vi "Starting Point.vi"() -> ()   [LabVIEW 2017]
uses:
  <vilib>/Analysis/baseanly.llb/Real A x B.vi
  <vilib>/Analysis/NI_AALBase.lvlib
  <vilib>/picture/3D Picture Control/NI_3D Picture Control.lvlib
panel:
  out "3D Picture":refnum<vi>(3d-picture)
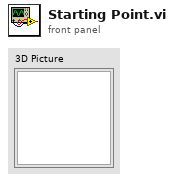
[diagram p1: front panel]
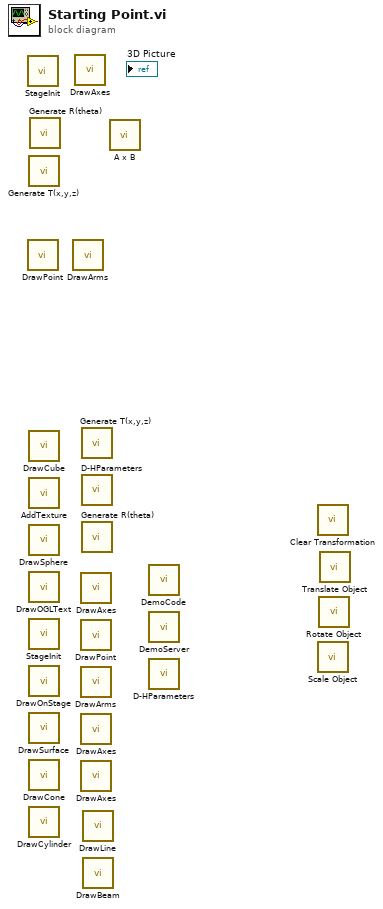
[diagram p0: block diagram]
diagram:
  n1 = call "StageInit.vi"() -> ()  [unwired: 4 in, 2 out]
  n2 = call "DrawPoint.vi"() -> ()  [unwired: 3 in, 1 out]
  n3 = call "Generate T(x,y,z).vi"() -> ()  [unwired: 3 in, 1 out]
  n4 = call "DrawCube.vi"() -> ()  [unwired: 6 in, 2 out]
  n5 = call "AddTexture.vi"() -> ()  [unwired: 4 in, 2 out]
  n6 = call "DrawSphere.vi"() -> ()  [unwired: 6 in, 2 out]
  n7 = call "DrawOGLText.vi"() -> ()  [unwired: 6 in, 2 out]
  n8 = call "StageInit.vi"() -> ()  [unwired: 4 in, 2 out]
  n9 = call "DrawOnStage.vi"() -> ()  [unwired: 3 in, 3 out]
  n10 = call "DrawSurface.vi"() -> ()  [unwired: 6 in, 2 out]
  n11 = call "DrawCone.vi"() -> ()  [unwired: 6 in, 2 out]
  n12 = call "DrawCylinder.vi"() -> ()  [unwired: 6 in, 2 out]
  n13 = call "Generate R(theta).vi"() -> ()  [unwired: 3 in, 1 out]
  n14 = call "DrawArms.vi"() -> ()  [unwired: 6 in, 2 out]
  n15 = call "DrawAxes.vi"() -> ()  [unwired: 5 in, 1 out]
  n16 = call "DrawAxes.vi"() -> ()  [unwired: 5 in, 1 out]
  n17 = call "DrawPoint.vi"() -> ()  [unwired: 3 in, 1 out]
  n18 = call "DrawArms.vi"() -> ()  [unwired: 6 in, 2 out]
  n19 = call "DrawAxes.vi"() -> ()  [unwired: 5 in, 1 out]
  n20 = call "DrawAxes.vi"() -> ()  [unwired: 5 in, 1 out]
  n21 = call "Generate T(x,y,z).vi"() -> ()  [unwired: 3 in, 1 out]
  n22 = call "D-HParameters.vi"() -> ()  [unwired: 3 in, 1 out]
  n23 = call "Generate R(theta).vi"() -> ()  [unwired: 3 in, 1 out]
  n24 = call "DrawLine.vi"() -> ()  [unwired: 5 in, 2 out]
  n25 = call "DrawBeam.vi"() -> ()  [unwired: 6 in, 1 out]
  n26 = call-poly <vilib>:"A x B.vi"() -> ()  [unwired: 2 in, 2 out]
  n27 = call "DemoCode.vi"() -> ()  [unwired: 12 in]
  n28 = call "DemoServer.vi"() -> ()  [unwired: 12 in]
  n29 = call "D-HParameters.vi"() -> ()  [unwired: 3 in, 1 out]
  n30 = call <vilib>:"Clear Transformation.vi"() -> ()  [unwired: 10 in, 2 out]
  n31 = call <vilib>:"Scale Object.vi"() -> ()  [unwired: 10 in, 2 out]
  n32 = call <vilib>:"Rotate Object.vi"() -> ()  [unwired: 10 in, 2 out]
  n33 = call <vilib>:"Translate Object.vi"() -> ()  [unwired: 10 in, 2 out]
